vi "queueWriterTest.vi"() -> ()   [LabVIEW 2013]
uses:
  control/payloadData.ctl
panel:
  in  "cmd":string
  out "watchDog":i32
  in  "send":bool
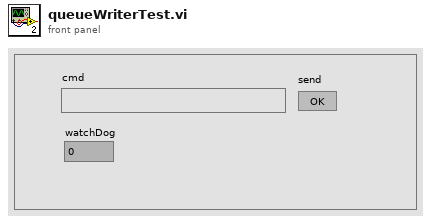
[diagram p1: front panel]
types:
  T1 = typedef "payloadData.ctl" = cluster{"Version":u32, "dataGramCount":i32, "cmd":string, "VariantData":variant}
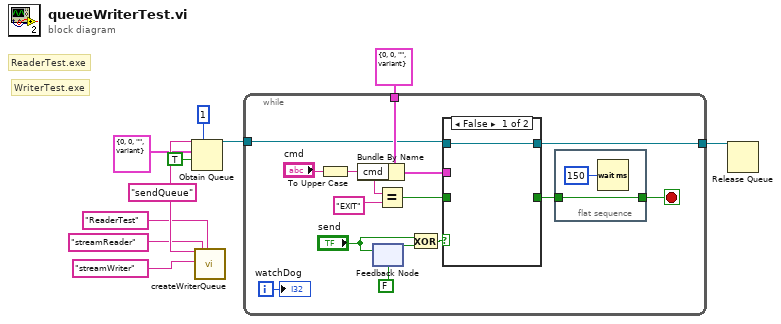
[diagram p0: block diagram]
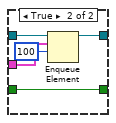
[diagram p2: hidden frame]
diagram:
  w9 = "sendQueue"
  # "WriterTest.exe"
  # "ReaderTest.exe"
  n1 = Obtain Queue(max queue size (-1, unlimited)=1, name (unnamed)=w9, element data type=T1 {"Version"=0, "dataGramCount"=0, "cmd"="", "VariantData"=variant} ("Data"), create if not found? (T)=TRUE) -> (queue out=w10:refnum<queue>)  [unwired: 1 in, 2 out]
  n2 = call "createWriterQueue.vi"("QueueName"=w9, "WriterEndPointName"="streamWriter" ("WriterName"), "ReaderEndPointName"="streamReader", "Remote application Name"="ReaderTest" ("ReaderEndPointName")) -> ()  [unwired: 15 in, 1 out]
  n3 = while {
    tunnel: w10 -> [w17]
    tunnel: T1 {"Version"=0, "dataGramCount"=0, "cmd"="", "VariantData"=variant} ("Data") -> [w25]
    tunnel: [w13] -> w3
    i -> [w23]
    stop <- w11 stop-if-true
    n4 = To Upper Case(1:"cmd") -> (0:w15:string)
    n5 = Bundle By Name(cluster=w25, "cmd"=w15) -> (w24:T1)
    n6 = feedback-in #1("send") -> ()
    n7 = feedback #1(FALSE ("send")) -> (w20:bool)
    n8 = Equal?(x=w15, y="EXIT") -> (x = y?=w14:bool)
    n9 = Exclusive Or(1:w20, 2:"send") -> (0:w19:bool)
    n10 = case shown="False" w19 {
      tunnel: w17 -> [w28 w33]
      tunnel: w24 -> [_ w32]
      tunnel: [w28 w31] -> w13
      tunnel: w14 -> [_ w30]
      tunnel: [_ w30] -> w12
      frame False {
      }
      frame True {
        n11 = Enqueue Element(queue=w33, element=w32, timeout in ms (-1)=100) -> (queue out=w31:refnum<queue>)  [unwired: 1 in, 2 out]
      }
    }
    n12 = flat-sequence {
      tunnel: w12 -> [w26]
      tunnel: [w26] -> w11
      frame #0 {
        n13 = Wait (ms)(milliseconds to wait=u32 150) -> ()  [unwired: 1 out]
      }
    }
    "watchDog" <- w23
  }
  n14 = Release Queue(queue=w3) -> ()  [unwired: 2 in, 3 out]
